vi "Train ramp.vi"(8 "Field":dbl[unit], 11 "Input":dbl[unit]) -> (0 "Change?":bool, 3 "Output":dbl[unit])   [LabVIEW 2009]
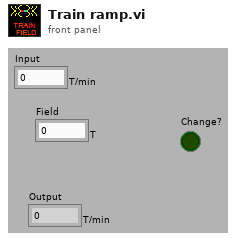
[diagram p1: front panel]
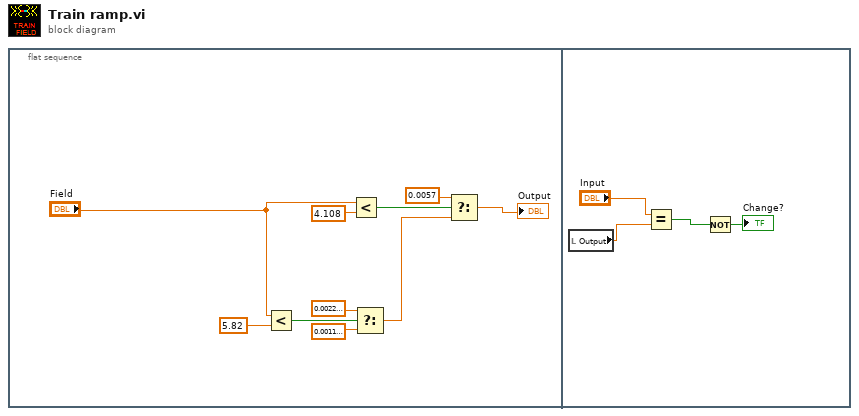
[diagram p0: block diagram]
diagram:
  n1 = flat-sequence {
    frame #0 {
      n2 = Less?(x="Field", y=dbl[unit] 5.82) -> (x < y?=w9:bool)
      n3 = Less?(x="Field", y=dbl[unit] 4.108) -> (x < y?=w3:bool)
      n4 = Select(t=dbl[unit] 0.0022833333333333334 ("y"), s=w9, f=dbl[unit] 0.0011333333333333334 ("y")) -> (s? t:f=w5:dbl[unit])
      n5 = Select(t=dbl[unit] 0.0057 ("y"), s=w3, f=w5) -> (s? t:f=→"Output":dbl[unit])
    }
    frame #1 {
      n6 = local read "Output"() -> (w14:dbl[unit])
      n7 = Equal?(x="Input", y=w14) -> (x = y?=w12:bool)
      n8 = Not(x=w12) -> (.not. x?=→"Change?":bool)
    }
  }
